vi "finishUp.vi"(8 "error in (no error)":errorcluster, 11 "SingleToneAction in":refnum<class "SingleToneAction.lvclass">) -> (0 "error out":errorcluster, 3 "SingleToneAction out":refnum<class "SingleToneAction.lvclass">)   [LabVIEW 2009, in "Views.lvlib" / "ScriptEditor.lvlib" / "SingleToneAction.lvclass"]
uses:
  SingleToneAction.lvclass
  SingleToneAction.lvclass/SingleToneAction.ctl
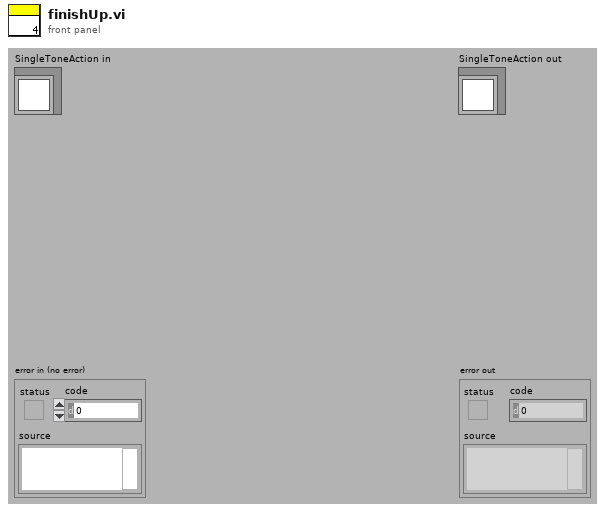
[diagram p1: front panel]
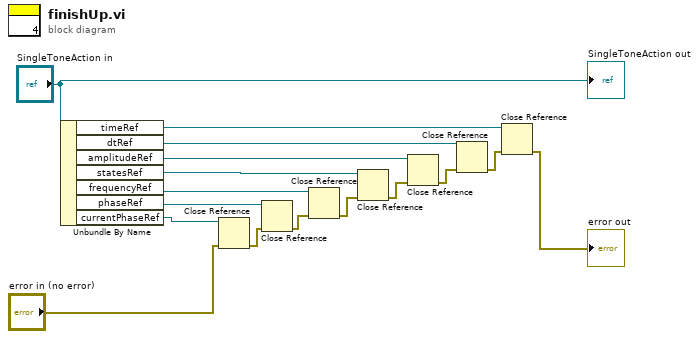
[diagram p0: block diagram]
diagram:
  n1 = Unbundle By Name("SingleToneAction in") -> ("timeRef"=w9:refnum<vi>, "dtRef"=w11:refnum<vi>, "amplitudeRef"=w12:refnum<vi>, "statesRef"=w15:refnum<vi>, "frequencyRef"=w16:refnum<vi>, "phaseRef"=w4:refnum<vi>, "currentPhaseRef"=w2:refnum<vi>)
  n2 = Close Reference(reference=w2, error in (no error)="error in (no error)") -> (error out=w3:errorcluster)
  n3 = Close Reference(reference=w4, error in (no error)=w3) -> (error out=w5:errorcluster)
  n4 = Close Reference(reference=w16, error in (no error)=w5) -> (error out=w14:errorcluster)
  n5 = Close Reference(reference=w15, error in (no error)=w14) -> (error out=w13:errorcluster)
  n6 = Close Reference(reference=w12, error in (no error)=w13) -> (error out=w10:errorcluster)
  n7 = Close Reference(reference=w11, error in (no error)=w10) -> (error out=w8:errorcluster)
  n8 = Close Reference(reference=w9, error in (no error)=w8) -> (error out=→"error out":errorcluster)
  "SingleToneAction out" <- "SingleToneAction in"
